vi "Part 2.vi"(11 "Input":string) -> (3 "Output":i64)   [LabVIEW 2021]
uses:
  <userlib>/_OpenG.lib/string/string.llb/Convert EOLs (String)__ogtk.vi
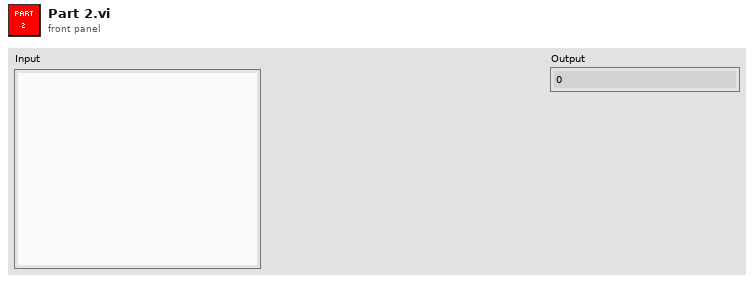
[diagram p1: front panel]
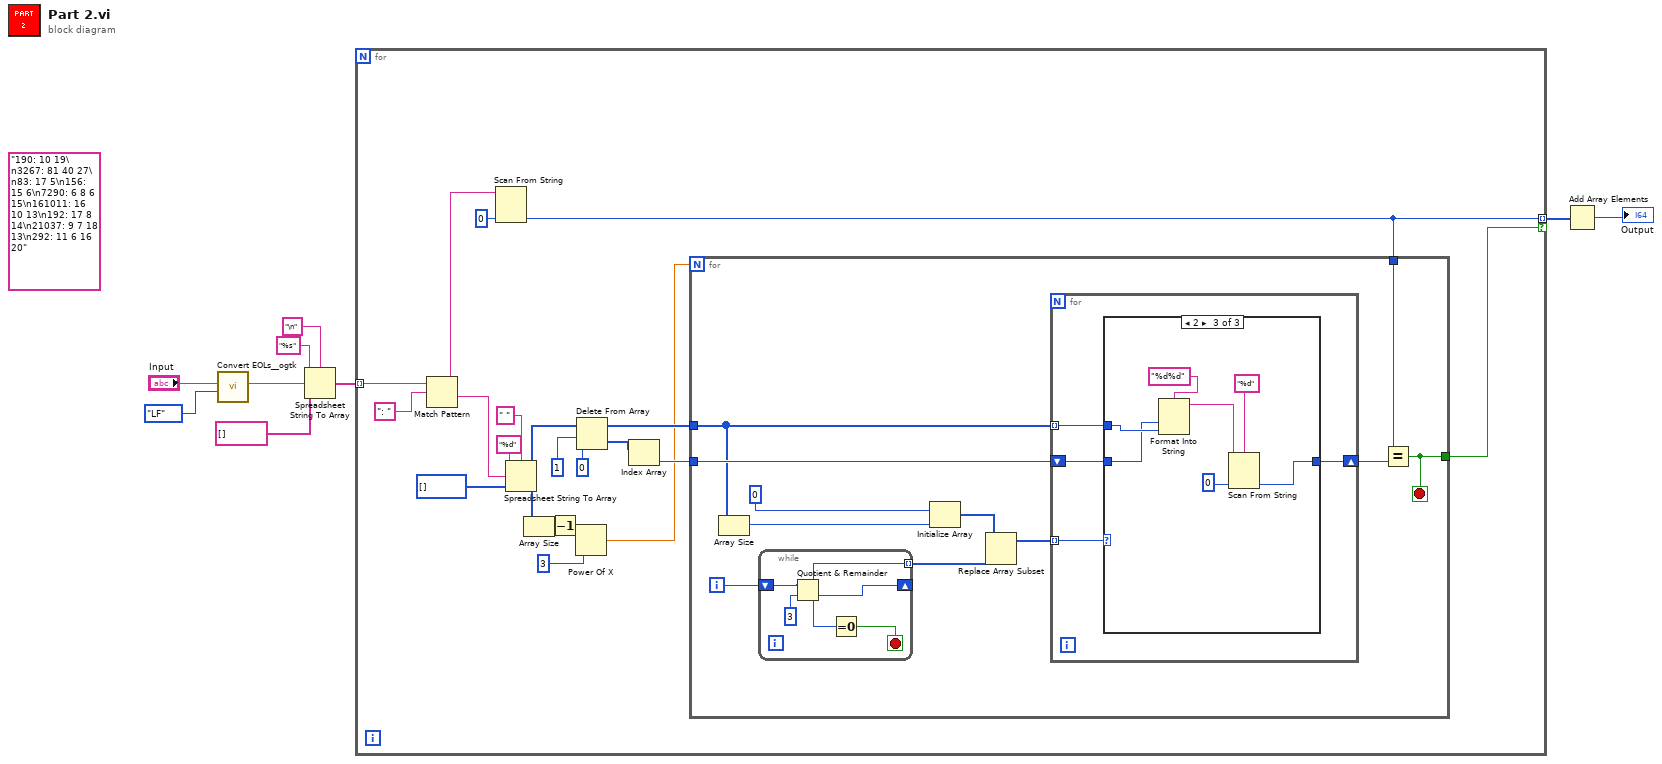
[diagram p0: block diagram]
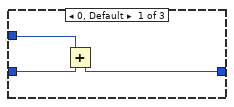
[diagram p2: hidden frame]
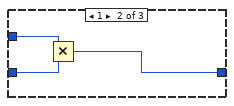
[diagram p3: hidden frame]
diagram:
  (unwired) "190: 10 19\n3267: 81 40 27\n83: 17 5\n156: 15 6\n7290: 6 8 6 15\n161011: 16 10 13\n192: 17 8 14\n21037: 9 7 18 13\n292: 11 6 16 20"
  n1 = call-poly <userlib>:"Convert EOLs__ogtk.vi"("Convert to:"=enum16{"CR", "LF", "CRLF"}."LF", "String in"="Input") -> ("String out"=w6:string)  [unwired: 9 in]
  n2 = Spreadsheet String To Array(delimiter (Tab)="\n", format string="%s", spreadsheet string=w6, array type (2D Dbl)=string[] []) -> (array=w4:string[])
  n3 = for {
    tunnel: w4 -> [w29] mode=indexing
    tunnel: [w15] -> w3 mode=indexing if=w14
    n4 = Match Pattern(string=w29, regular expression=": " ("delimiter (Tab)")) -> (before substring=w27:string, after substring=w26:string)  [unwired: 1 in, 2 out]
    n5 = Scan From String(input string=w27, default 1=i64 0) -> (output 1=w15:i64)  [unwired: 3 in, 3 out]
    n6 = Spreadsheet String To Array(delimiter (Tab)=" ", format string="%d", spreadsheet string=w26, array type (2D Dbl)=i64[] []) -> (array=w21:i64[])
    n7 = Array Size(array=w21) -> (size(s)=w11:i32)
    n8 = Decrement(x=w11) -> (x-1=w10:i32)
    n9 = Power Of X(1:3, 2:w10) -> (0:w12:dbl)
    n10 = Delete From Array(array=w21, length=1, index=0) -> (deleted portion=w17:i64[], array with subset deleted=w18:i64[])
    n11 = Index Array(array=w17) -> (element=w16:i64)  [unwired: 1 in]
    n12 = for {
      N: w12 -> [_]
      tunnel: w18 -> [w36]
      tunnel: w16 -> [w40]
      tunnel: w15 -> [w38]
      tunnel: [w37] -> w14
      i -> [w31]
      stop <- w37 stop-if-true
      n13 = Array Size(array=w36) -> (size(s)=w35:i32)
      n14 = while {
        shift-right: [w42] -> _
        shift-left: w31 -> [w45]
        tunnel: [w41] -> w30 mode=indexing
        stop <- w44 stop-if-true
        n15 = Quotient & Remainder(x=w45, y=3) -> (x-y*floor(x/y)=w41:i32, floor(x/y)=w42:i32)
        n16 = Equal To 0?(x=w42) -> (x = 0?=w44:bool)
      }
      n17 = Initialize Array(0, w35) -> (w33:i32[])
      n18 = Replace Array Subset(array=w33, new element=w30) -> (w32:i32[])  [unwired: 1 in]
      n19 = for {
        tunnel: w36 -> [w47] mode=indexing
        shift-right: [w46] -> w39
        shift-left: w40 -> [w48]
        tunnel: w32 -> [w49] mode=indexing
        n20 = case shown="2" w49 {
          tunnel: w48 -> [w52 w55 w56]
          tunnel: w47 -> [w51 w54 w57]
          tunnel: [w50 w53 w60] -> w46
          frame 0, Default {
            n21 = Add(x=w51, y=w52) -> (x+y=w50:i64)
          }
          frame 1 {
            n22 = Multiply(x=w54, y=w55) -> (x*y=w53:i64)
          }
          frame 2 {
            n23 = Format Into String(format string="%d%d", w56, w57) -> (resulting string=w62:string)  [unwired: 2 in, 1 out]
            n24 = Scan From String(format string="%d", input string=w62, default 1=i64 0) -> (output 1=w60:i64)  [unwired: 2 in, 3 out]
          }
        }
      }
      n25 = Equal?(x=w38, y=w39) -> (x = y?=w37:bool)
    }
  }
  n26 = Add Array Elements(numeric array=w3) -> (sum=→"Output":i64)
